vi "Get General Configuration.vi"(8 "error in (no error)":errorcluster, 11 "Ethernet in":refnum<class "ENET_BS1200.lvclass">) -> (0 "error out":errorcluster, 1 "Configuration Error?":bool, 2 "Protocol":T1, 3 "Ethernet out":refnum<class "ENET_BS1200.lvclass">, 4 "Cell Inhibit Enable":bool)   [LabVIEW 2021, in "BS120x Driver.lvlib" / "ENET_BS1200.lvclass"]
doc: "Retrieve Battery Simulator 1200 general settings.\n(c) 2019 Bloomy Controls, Inc. All rights reserved."
uses:
  ENET_BS1200.lvclass
  TypeDefs/Protocol.ctl
  <vilib>/WebDAVClient/Advanced/Get Buffer.vi
  ENET_BS1200.lvclass/ENET_BS1200.ctl
  <vilib>/WebDAVClient/NI_WebDAV.lvlib
  BS120x.lvclass
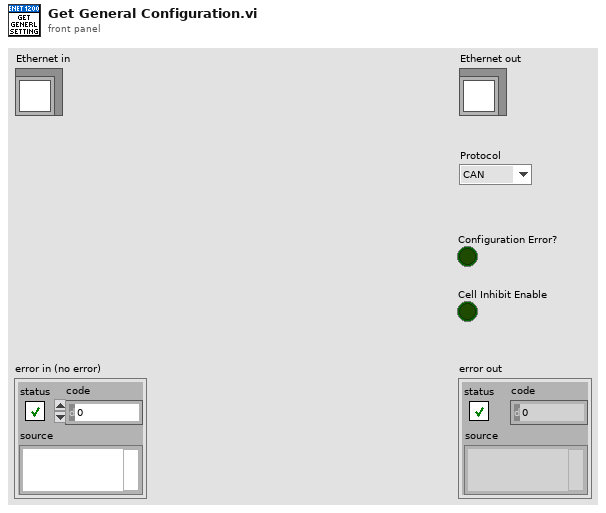
[diagram p1: front panel]
types:
  T1 = typedef "BS120x Driver.lvlib/BS120x.lvclass/Protocol.ctl" = enum16{"CAN", "Ethernet"}
  T2 = typedef "NI_WebDAV.lvlib/SessionHandle.ctl" = refnum<k1>
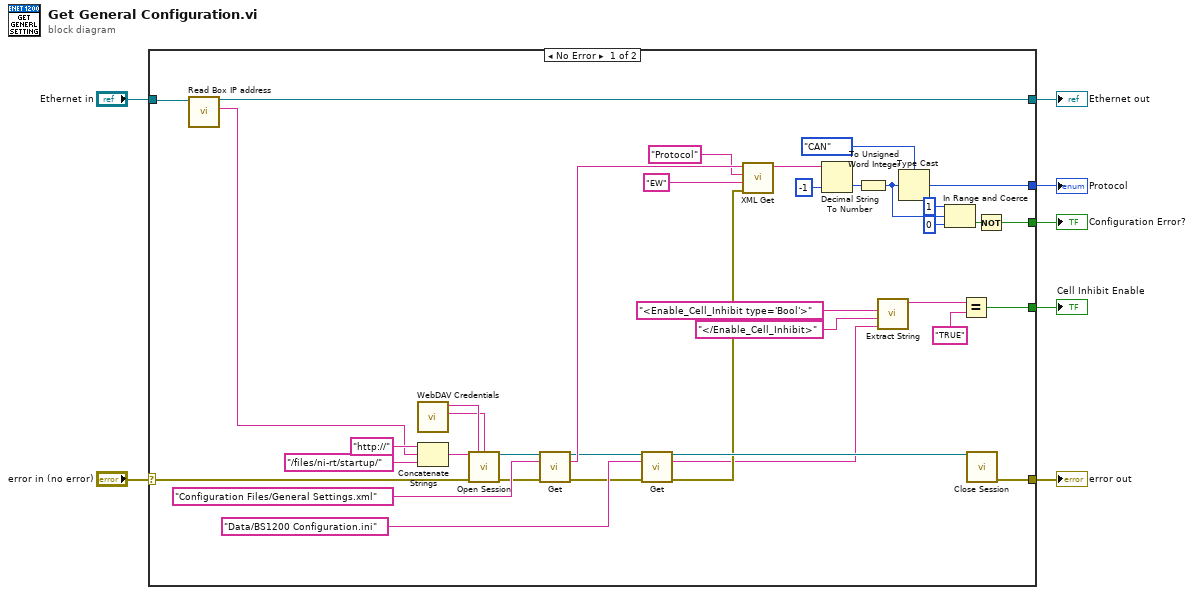
[diagram p0: block diagram]
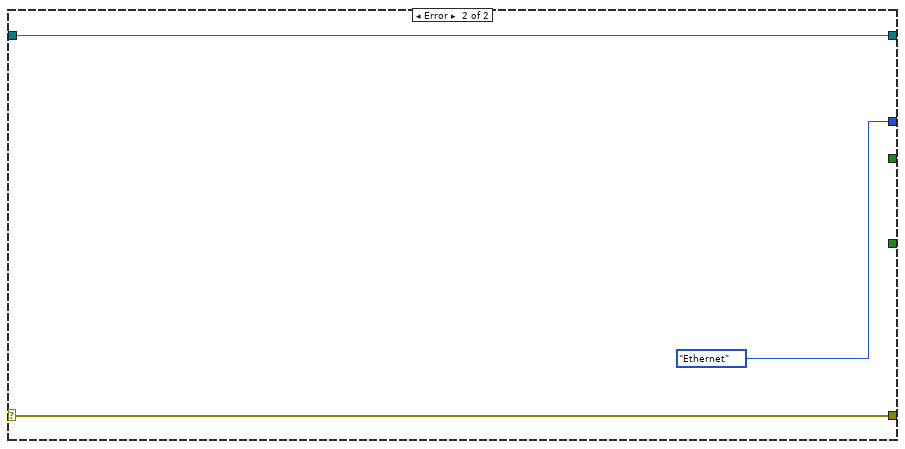
[diagram p2: hidden frame]
diagram:
  n1 = case shown="No Error" "error in (no error)" {
    selector: "error in (no error)" -> [w42 w47]
    tunnel: [w33 w47] -> w6
    tunnel: [w21 w46] -> w4
    tunnel: "Ethernet in" -> [w22 w46]
    tunnel: [w24 _] -> w3
    tunnel: [w20 Protocol."Ethernet" ("Protocol")] -> w2
    tunnel: [w8 _] -> w1
    frame No Error {
      n2 = call-dynamic "Read Box IP address.vi"("ENET_BS120x in"=w22) -> ("Box IP address"=w19:string, "ENET_BS120x out"=w21:refnum<class "ENET_BS1200.lvclass">)  [unwired: 8 in, 1 out]
      n3 = call "WebDAV Credentials.vi"() -> ("Password"=w40:string, "Username"=w41:string)  [unwired: 10 in]
      n4 = Concatenate Strings("http://" ("string"), w19, "/files/ni-rt/startup/" ("string")) -> (w39:string)
      n5 = call <vilib>:"Open Session.vi"("host uri prefix"=w39, "username"=w41, "password"=w40, "error in (no error)"=w42) -> ("session handle out"=w32:T2, "error out"=w31:errorcluster)  [unwired: 10 in]
      n6 = call-poly <vilib>:"Get.vi"("session handle"=w32, "relative uri"="Configuration Files/General Settings.xml" ("string"), "error in (no error)"=w31) -> ("session handle out"=w18:T2, "data"=w37:string, "error out"=w15:errorcluster)  [unwired: 10 in]
      n7 = call-poly <vilib>:"Get.vi"("session handle"=w18, "relative uri"="Data/BS1200 Configuration.ini", "error in (no error)"=w15) -> ("session handle out"=w17:T2, "data"=w11:string, "error out"=w14:errorcluster)  [unwired: 10 in]
      n8 = call "XML Get.vi"("error in (no error)"=w14, "Data Type"="EW" ("regular expression"), "Parameter"="Protocol" ("regular expression"), "XML String in"=w37) -> ("Value"=w23:string)  [unwired: 6 in, 1 out]
      n9 = Decimal String To Number(string=w23, default (0L)=-1 ("default (0 I32)")) -> (number=w29:i32)  [unwired: 1 in, 1 out]
      n10 = To Unsigned Word Integer(number=w29) -> (unsigned 16bit integer=w28:u16)
      n11 = call "Extract String.vi"("Input String"=w11, "Text After String"="</Enable_Cell_Inhibit>", "Text Before String"="<Enable_Cell_Inhibit type='Bool'>") -> ("Value String"=w10:string)  [unwired: 8 in]
      n12 = Type Cast(type=Protocol."CAN" ("Protocol"), x=w28) -> (*(type *) &x=w20:T1)
      n13 = In Range and Coerce(upper limit=u16 1, x=w28, lower limit=u16 0) -> (In Range?=w25:bool)  [unwired: 1 out]
      n14 = Equal?(x=w10, y="TRUE") -> (x = y?=w8:bool)
      n15 = call <vilib>:"Close Session.vi"("session handle"=w17) -> ("error out"=w33:errorcluster)  [unwired: 14 in]
      n16 = Not(x=w25) -> (.not. x?=w24:bool)
    }
    frame Error {
    }
  }
  "error out" <- w6
  "Ethernet out" <- w4
  "Protocol" <- w2
  "Configuration Error?" <- w3
  "Cell Inhibit Enable" <- w1
